vi "Remove.vi"(8 "error in (no error)":errorcluster, 11 "ID":i32) -> (0 "error out":errorcluster, 3 "Module":T1)   [LabVIEW 2018, in "Core.lvlib" / "Module.lvlib"]
uses:
  Module.lvlib
  Controls/Module.ctl
  Controls/Instance.ctl
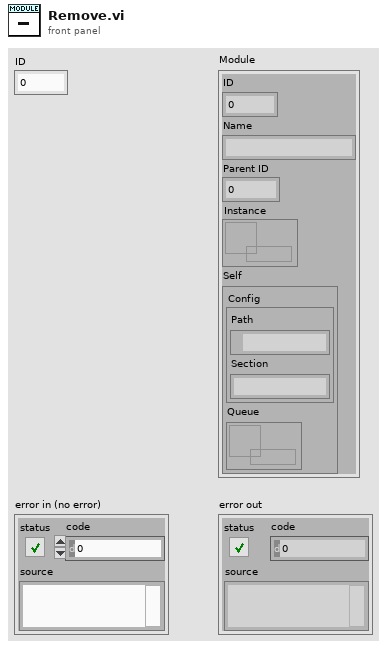
[diagram p1: front panel]
types:
  T1 = typedef "Core.lvlib/Module.lvlib/Module.ctl" = cluster{"ID":i32, "Name":string, "Parent ID":i32, "Instance":refnum<data-value>, "Self":T2}
  T2 = typedef "Core.lvlib/Module.lvlib/Instance.ctl" = cluster{"Config":cluster{"Path":path, "Section":string}, "Queue":refnum<queue>}
  T3 = cluster{"ID":i32, "Name":string, "Parent ID":i32, "Instance":refnum<data-value>}[]
  T4 = cluster{"ID":i32, "Name":string, "Parent ID":i32, "Instance":refnum<data-value>}
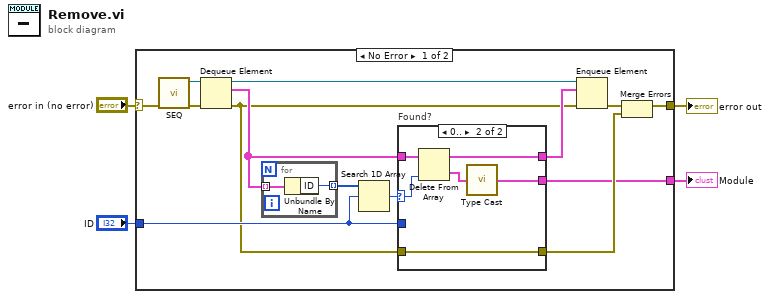
[diagram p0: block diagram]
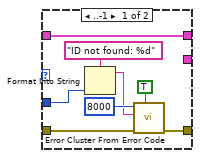
[diagram p2: hidden frame]
diagram:
  n1 = case shown="No Error" "error in (no error)" {
    selector: "error in (no error)" -> [w18 w35]
    tunnel: "ID" -> [w10 _]
    tunnel: [w8 w35] -> w2
    tunnel: [w12 _] -> w1
    frame No Error {
      n2 = call "SEQ.vi"("error in (no error)"=w18) -> ("error out"=w17:errorcluster, "Modules"=w16:refnum<queue>)  [unwired: 8 in, 1 out]
      n3 = Dequeue Element(queue=w16, error in (no error)=w17) -> (queue out=w9:refnum<queue>, element=w14:T3, error out=w5:errorcluster)  [unwired: 1 in, 1 out]
      n4 = for {
        tunnel: w14 -> [w20] mode=indexing
        tunnel: [w19] -> w15 mode=indexing
        n5 = Unbundle By Name(w20) -> ("ID"=w19:i32)
      }
      n6 = Search 1D Array(1D array=w15, element=w10) -> (index of element=w11:i32)  [unwired: 1 in]
      n7 = case "Found?" shown="0.." w11 {
        selector: w11 -> [_ w31]
        tunnel: w14 -> [w21 w34]
        tunnel: w5 -> [w28 w29]
        tunnel: [w27 w29] -> w13
        tunnel: [_ w32] -> w12
        tunnel: w10 -> [w24 _]
        tunnel: [w21 w30] -> w6
        frame ..-1 {
          n8 = Format Into String(format string="ID not found: %d", w24) -> (resulting string=w22:string)  [unwired: 2 in, 1 out]
          n9 = call <vilib>:"Error Cluster From Error Code.vi"("show call chain? (False)"=TRUE, "error in (no error)"=w28, "error message (\"\")"=w22, "error code (0)"=8000) -> ("error out"=w27:errorcluster)  [unwired: 5 in]
        }
        frame 0.. {
          n10 = Delete From Array(array=w34, index=w31) -> (deleted portion=w33:T4, array with subset deleted=w30:T3)  [unwired: 1 in]
          n11 = call "Type Cast.vi"("Module in"=w33) -> ("Module"=w32:T1)
        }
      }
      n12 = Enqueue Element(queue=w9, element=w6, error in (no error)=w5) -> (error out=w7:errorcluster)  [unwired: 1 in, 2 out]
      n13 = Merge Errors(w7, w13) -> (w8:errorcluster)
    }
    frame Error {
    }
  }
  "error out" <- w2
  "Module" <- w1
